vi "CalcularTiempo.vi"(9 "20xResolucion":dbl format="%#_13g", 10 "NPS Aplicado":string[](array[string]), 11 "Frecuencias":string[](array[string])) -> (3 "Tiempo":string[](array[string]))   [LabVIEW 2019, in "Prueba33.lvclass"]
uses:
  Prueba33.lvclass
panel:
  out "Tiempo (s)":dbl
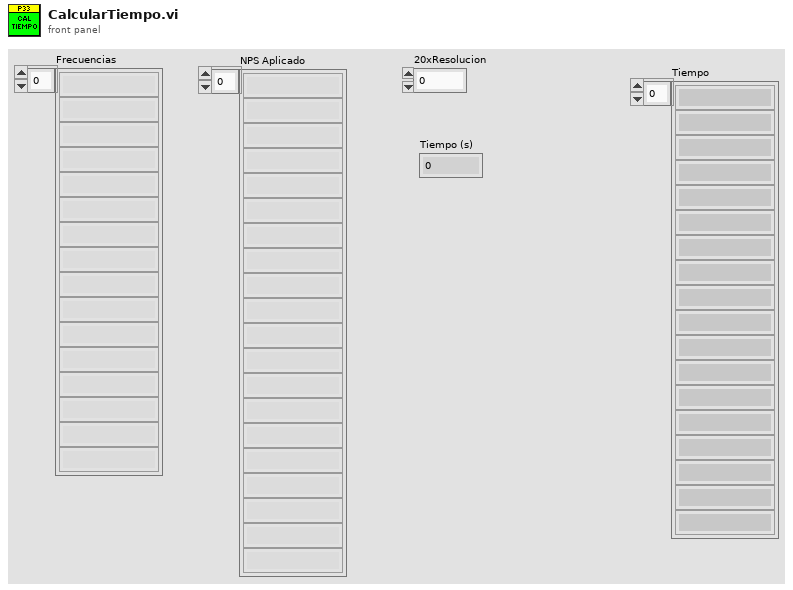
[diagram p1: front panel]
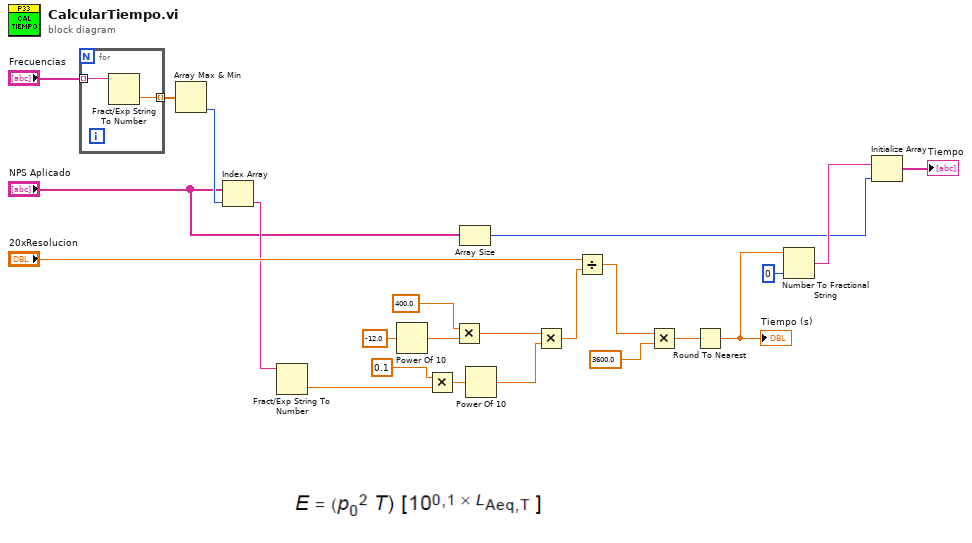
[diagram p0: block diagram]
diagram:
  n1 = for {
    tunnel: "Frecuencias" -> [w25] mode=indexing
    tunnel: [w24] -> w10 mode=indexing
    n2 = Fract/Exp String To Number(string=w25) -> (number=w24:dbl)  [unwired: 3 in, 1 out]
  }
  n3 = Array Max & Min(array=w10) -> (min index (indices)=w9:i32)  [unwired: 3 out]
  n4 = Index Array(array="NPS Aplicado", index=w9) -> (element=w8:string)
  n5 = Fract/Exp String To Number(string=w8) -> (number=w7:dbl)  [unwired: 3 in, 1 out]
  n6 = Power Of 10(x=-12.0) -> (10^x=w12:dbl)
  n7 = Multiply(x=0.1, y=w7) -> (x*y=w18:dbl)
  n8 = Multiply(x=400.0, y=w12) -> (x*y=w20:dbl)
  n9 = Array Size(array="NPS Aplicado") -> (size(s)=w2:i32)
  n10 = Power Of 10(x=w18) -> (10^x=w17:dbl)
  n11 = Multiply(x=w20, y=w17) -> (x*y=w16:dbl)
  n12 = Divide(x="20xResolucion", y=w16) -> (x/y=w15:dbl)
  n13 = Multiply(x=w15, y=3600.0) -> (x*y=w13:dbl)
  n14 = Round To Nearest(number=w13) -> (nearest integer value=w6:dbl)
  "Tiempo (s)" <- w6
  n15 = Number To Fractional String(number=w6, precision (6)=i16 0) -> (F-format string=w3:string)  [unwired: 2 in]
  n16 = Initialize Array(w3, w2) -> (→"Tiempo":string[])
